vi "Write Abort.vi"(8 "error in (no error)":errorcluster, 10 "Abort value":bool, 11 "Guardian in":refnum<class "Guardian.lvclass">) -> (0 "error out":errorcluster, 3 "Guardian out":refnum<class "Guardian.lvclass">)   [LabVIEW 2026, in "TALOS.lvlib" / "Guardian.lvlib" / "Guardian.lvclass"]
doc: "Single point of writing access to Abort.\nMinimises race conditions, and it's easier to understand where Abort is written."
uses:
  Guardian.lvclass
  Guardian.lvclass/Guardian.ctl
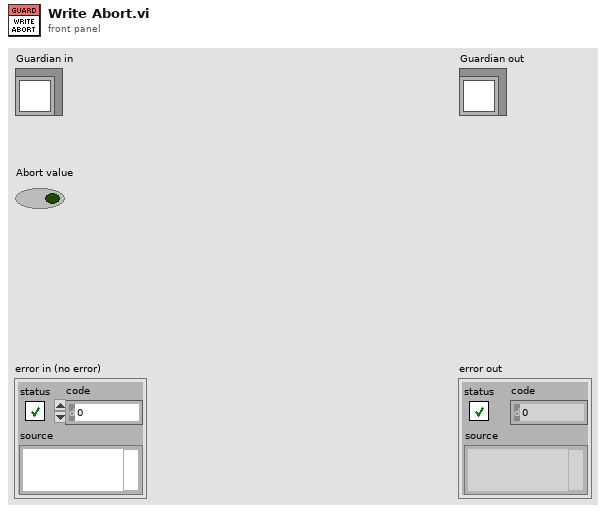
[diagram p1: front panel]
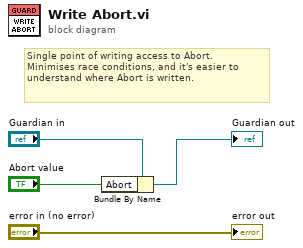
[diagram p0: block diagram]
diagram:
  # "Single point of writing access to Abort.\nMinimises race conditions, and it's easier to understand where Abort is written."
  n1 = Bundle By Name(cluster="Guardian in", "Abort"="Abort value") -> (→"Guardian out":refnum<class "Guardian.lvclass">)
  "error out" <- "error in (no error)"
